vi "LCfiletransfer.vi"() -> ()   [LabVIEW 2018]
panel:
  in  "Filename":string
  in  "File Directory":path
  out "File data":string
  out "error out":errorcluster
  out "VISA resource name out":refnum<visa-resource-name>
  in  "Source Filename":string
  in  "error in (no error)":errorcluster
  in  "VISA resource name":refnum<visa-resource-name>
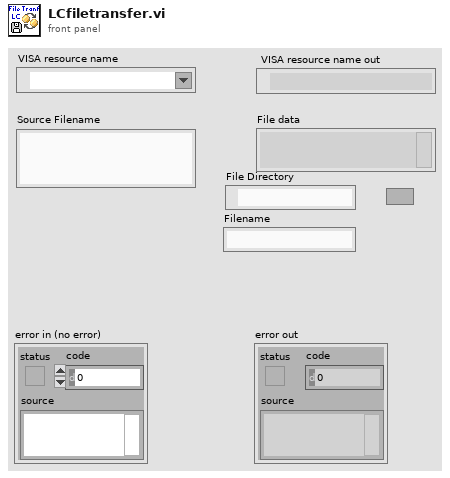
[diagram p1: front panel]
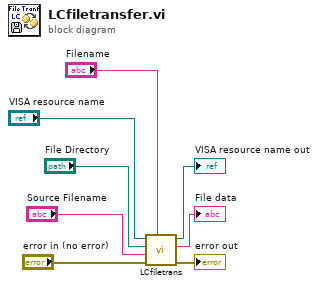
[diagram p0: block diagram]
diagram:
  n1 = call "LCfiletrans.vi"("Filename"="Filename", "error in (no error)"="error in (no error)", "Source Filename"="Source Filename", "File Directory"="File Directory", "VISA Refnum in"="VISA resource name") -> ("error out"=→"error out":errorcluster, "File data"=→"File data":string, "VISA Refnum out"=→"VISA resource name out":refnum<visa-resource-name>)  [unwired: 4 in]
